vi "Circle_Setting_UI.vi"(6 "Analysis_Setting IN":T2={"PreProcess"=enum."*Algorithm*", "Parameter"=""}, 8 "error in (no error)":errorcluster, 9 "ProjectName":string, 10 "ROI List IN":refnum<vi>, 11 "Vision_Image":T11(plugin-control)) -> (0 "error out":errorcluster, 1 "Cancel?":bool, 3 "Analysis_Setting":T2={"PreProcess"=enum."*Algorithm*", "Parameter"=""})   [LabVIEW 2019]
uses:
  <vilib>/userdefined/High Color/IMAQdx.ctl
  <vilib>/vision/NI_Vision_Development_Module.lvlib
  Controls/Analysis_Type.ctl
  Controls/Analysis_Setting.ctl
  Controls/_UI Command Cluster/Circle_UI Command Cluster.ctl
  <vilib>/vision/Measure.llb/Edge Polarity.ctl
  <vilib>/vision/Measure.llb/Edge Options.ctl
  Controls/Circle/Analysis_Circle_Parameter.ctl
  Controls/V_Analysis_Type.ctl
  Ctrl/VisionProcessName.ctl
panel:
  in  "Snap?":bool
  in  "ROI Descriptor":T1
  out "Numeric":i32
  in  "Done":bool
  in  "Clamp_UI Command":T4(ring)
  in  "Cancel":bool
  in  "ClampTab":T5(tab)
  in  "Options":T8={"Search  Direction"=0, "Edge Options"={"Edge Polarity"=0, "Kernel Size"=3, "Width"=3, "Minimum Edge Strength"=10.0, "Interpolation Type"=enum."Bilinear Fixed", "Data Processing Method"=enum."Average"}, "Show Search Area"=FALSE, "Show Search Lines"=FALSE, "Show Edges Found"=FALSE, "Show Result"=TRUE, "Search Area Color"=65280, "Search Lines Color"=255, "Edge Locations Color"=16776960, "Result Color"=16711680, "Overlay Group Name"=""} {"Search  Direction" items=["Outside to Inside", "Inside to Outside"]; "Edge Options"."Edge Polarity" items=["All Edges", "Rising Edges", "Falling Edges"]; "Edge Options"."Minimum Edge Strength" format="%.2f"; "Edge Options"."Width" step=2; "Edge Options"."Kernel Size" step=2}
  in  "Circle Fit Options":T9={"Process"=enum."Get First Edge", "Step Size"=3.0, "Max Pixel Radius"=3}
  out "Fitted Circle":T10 {"Average SNR (dB)" format="%.2f"; "Average Strength" format="%.2f"; "Roundness (Real-World)" format="%.2f"; "Radius (Real-World)" format="%.2f"; "Center (Real-World)"."Y" format="%.2f"; "Center (Real-World)"."X" format="%.2f"; "Radius (Pixels)" format="%.2f"; "Center (Pixels)"."Y" format="%.2f"; "Center (Pixels)"."X" format="%.2f"}
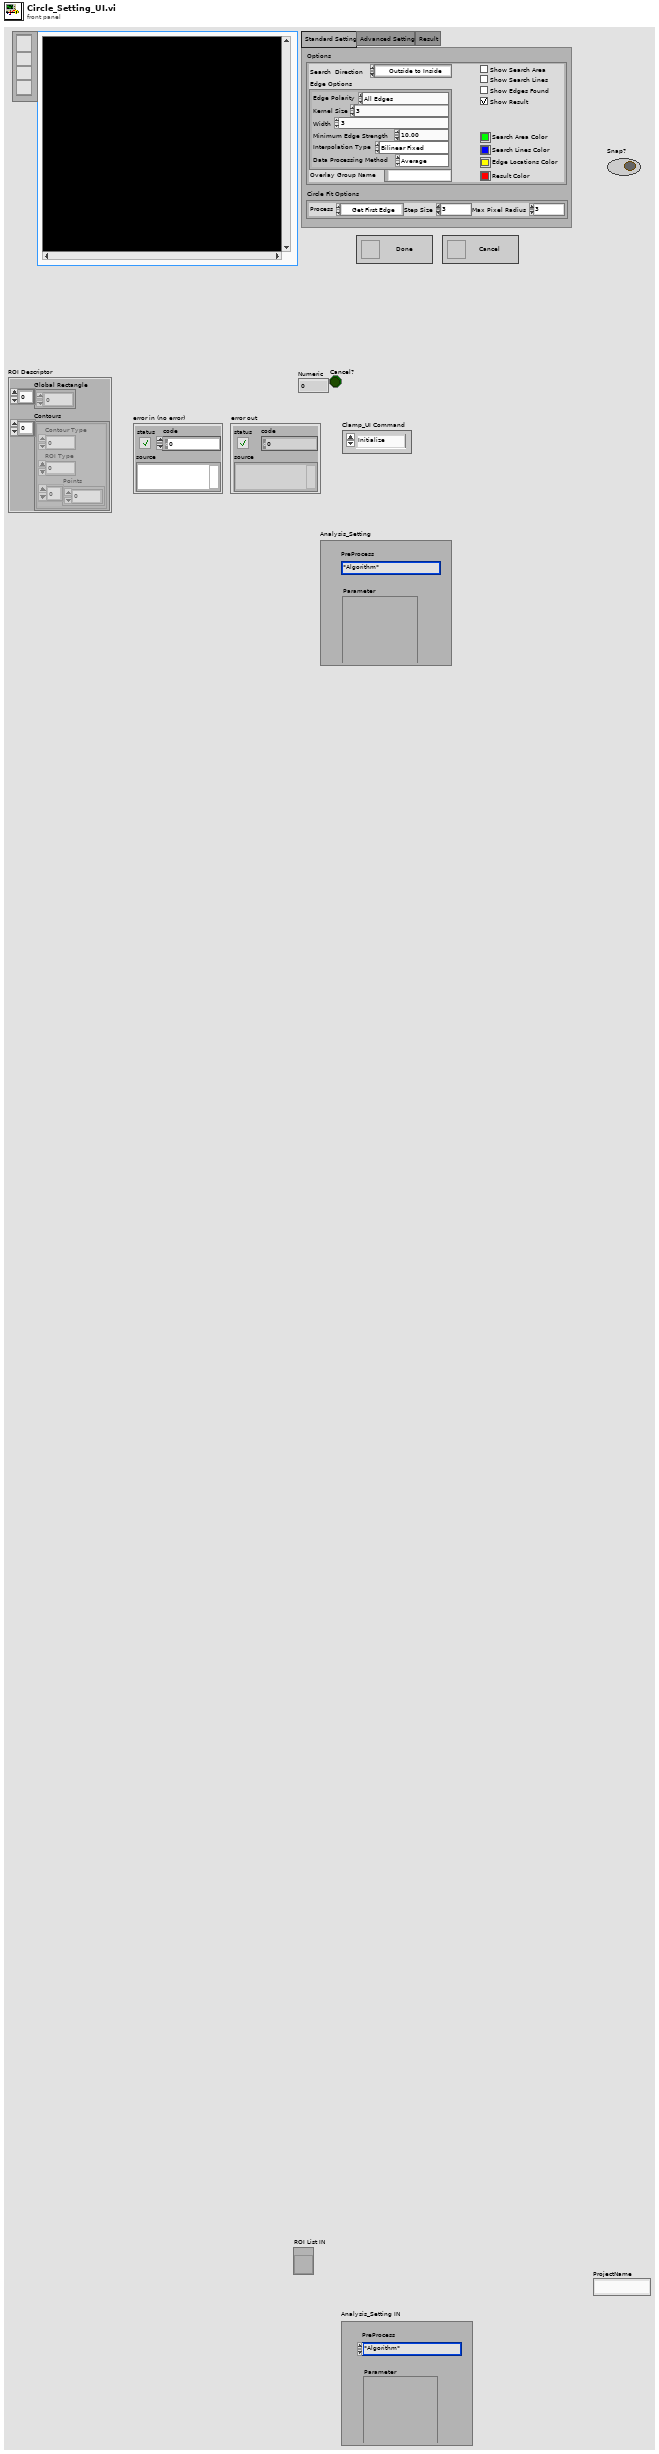
[diagram p1: front panel]
types:
  T1 = cluster{"Global Rectangle":i32[], "Contours":cluster{"Contour Type":u32, "ROI Type":u32, "Points":i32[]}[]}
  T2 = typedef "Analysis_Setting.ctl" = cluster{"PreProcess":T3, "Parameter":string}
  T3 = typedef "VisionProcessName.ctl" = enum16{"*CamParameter*", "CamAttributes", "*Preprocess*", "CG_Brightness", "C_Plane Extraction", "C_Threshold", "G_Lookup Table", "G_Threshold", "B_Image Inversion", "*Algorithm*", "CG_Histogram", "C_Color Matching", "C_Color Pattern Matching", "G_PatternMatch", "CG_Find Straight Edge", "CG_Adv. Find Straight Edge", "CG_Find Circular Edge", "G_Max Clamp", "G_Clamp (Rake)", "G_Pattern Matching"}
  T4 = enum16{"Initialize", "Done", "Run Algorithm", "Cancel"}
  T5 = enum32{"Standard Setting", "Advanced Setting", "Result"}
  T6 = typedef "Edge Options.ctl" = cluster{"Edge Polarity":T7, "Kernel Size":u32, "Width":u32, "Minimum Edge Strength":sgl, "Interpolation Type":enum32{"Zero Order", "Bilinear", "Quadratic", "Cubic", "Bilinear Fixed"}, "Data Processing Method":enum32{"Average", "Median"}}
  T7 = typedef "Edge Polarity.ctl" = u32
  T8 = cluster{"Search  Direction":u32, "Edge Options":T6, "Show Search Area":bool, "Show Search Lines":bool, "Show Edges Found":bool, "Show Result":bool, "Search Area Color":u32, "Search Lines Color":u32, "Edge Locations Color":u32, "Result Color":u32, "Overlay Group Name":string}
  T9 = cluster{"Process":enum16{"Get First Edge", "Get First + Last Edge", "Get All Edges", "Get Best Edge"}, "Step Size":dbl, "Max Pixel Radius":i32}
  T10 = cluster{"Center (Pixels)":cluster{"X":sgl, "Y":sgl}, "Radius (Pixels)":dbl, "Center (Real-World)":cluster{"X":sgl, "Y":sgl}, "Radius (Real-World)":dbl, "Roundness (Real-World)":dbl, "Average Strength":dbl, "Average SNR (dB)":dbl}
  T11 = typedef "IMAQ Image.ctl" = refnum<image>
  T12 = typedef "Circle_UI Command Cluster.ctl" = cluster{"Circle_UI Command":enum16{"Initialize", "Done", "Run Algorithm", "Cancel"}, "Snap Simulation Mouse Down":bool, "ROI Descriptor":cluster{"Global Rectangle":i32[], "Contours":cluster{"Contour Type":u32, "ROI Type":u32, "Points":i32[]}[]}, "Options":cluster{"Search  Direction":u32, "Edge Options":T6, "Show Search Area":bool, "Show Search Lines":bool, "Show Edges Found":bool, "Show Result":bool, "Search Area Color":u32, "Search Lines Color":u32, "Edge Locations Color":u32, "Result Color":u32, "Overlay Group Name":string}, "Circle Fit Options":cluster{"Process":enum16{"Get First Edge", "Get First + Last Edge", "Get All Edges", "Get Best Edge"}, "Step Size":dbl, "Max Pixel Radius":i32}}
  T13 = typedef "IMAQ Line" = cluster{"Start X":i32, "Start Y":i32, "End X":i32, "End Y":i32}
  T14 = typedef "IMAQdx.ctl" = refnum<k21>
  T15 = cluster{"Contour Type":u32, "ROI Type":u32, "Points":i32[]}
  T16 = typedef "Image Type" = u32
  T17 = typedef "Analysis_Type.ctl" = u16
  T18 = typedef "Analysis_Circle_Parameter.ctl" = cluster{"ROI Descriptor":cluster{"Global Rectangle":i32[], "Contours":cluster{"Contour Type":u32, "ROI Type":u32, "Points":i32[]}[]}, "Options":cluster{"Search  Direction":u32, "Edge Options":T6, "Show Search Area":bool, "Show Search Lines":bool, "Show Edges Found":bool, "Show Result":bool, "Search Area Color":u32, "Search Lines Color":u32, "Edge Locations Color":u32, "Result Color":u32, "Overlay Group Name":string}, "Circle Fit Options":cluster{"Process":enum16{"Get First Edge", "Get First + Last Edge", "Get All Edges", "Get Best Edge"}, "Step Size":dbl, "Max Pixel Radius":i32}}
  T19 = typedef "ROI Descriptor" = cluster{"Global Rectangle":i32[], "Contours":cluster{"ID":enum32{"External", "Internal"}, "Type":u32, "Coordinates":i32[]}[]}
  T20 = typedef "Analysis_Setting.ctl" = cluster{"PreProcess":T21, "Parameter":string}
  T21 = typedef "V_Analysis_Type.ctl" = enum16{"None", "C_Color Pattern Matching", "G_PatternMatching", "G_ShapeDectect", "G_GeometricMatch", "B_Area Check"}
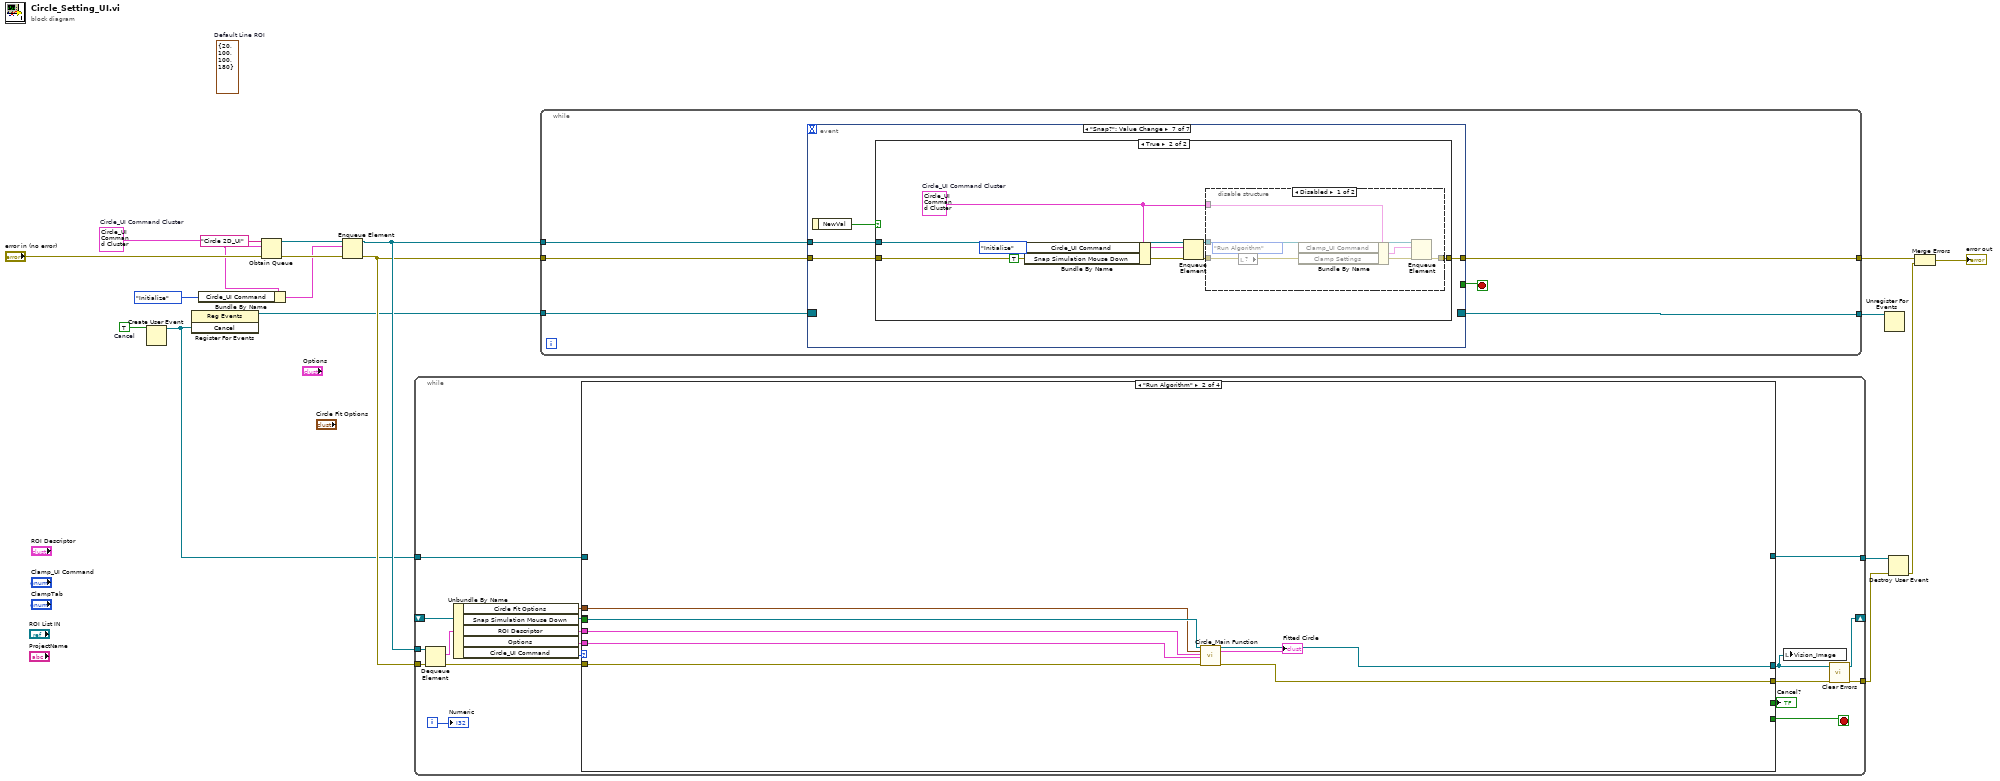
[diagram p0: block diagram]
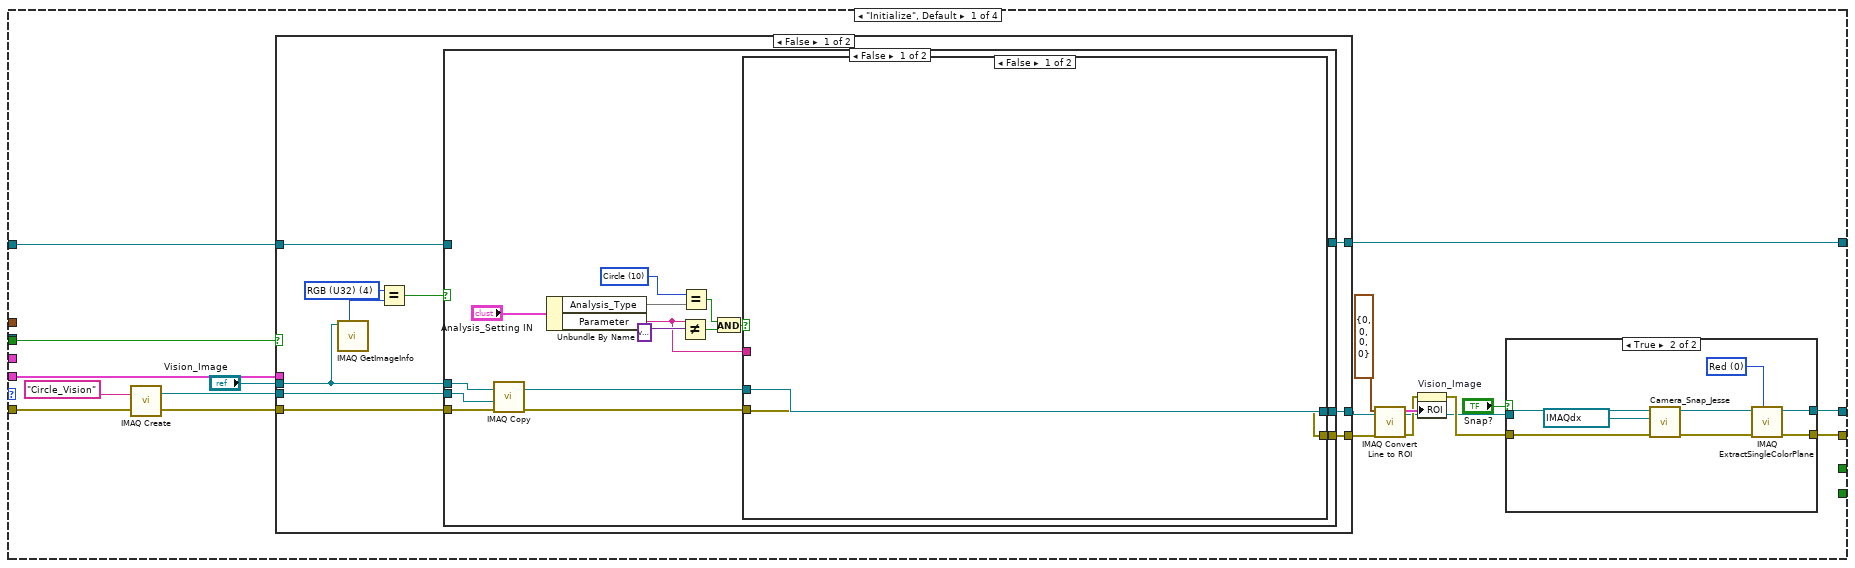
[diagram p2: hidden frame]
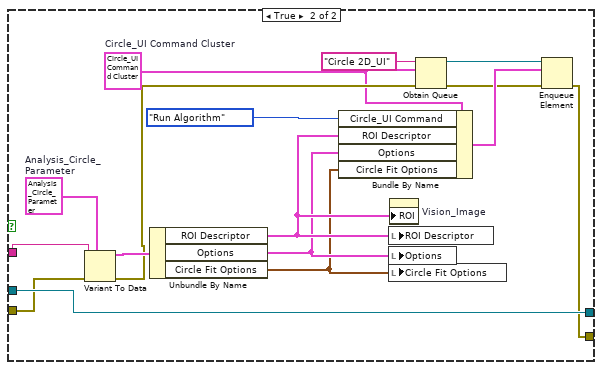
[diagram p4: hidden frame]
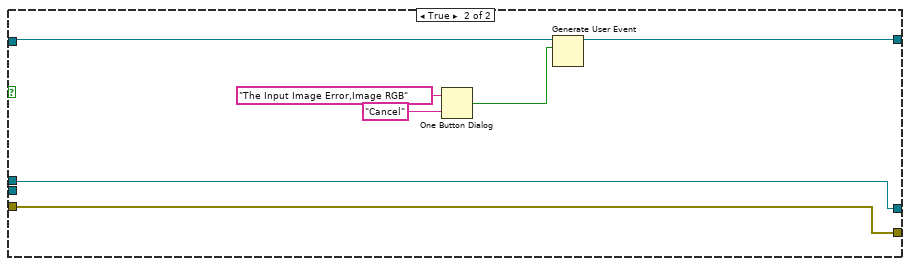
[diagram p5: hidden frame]
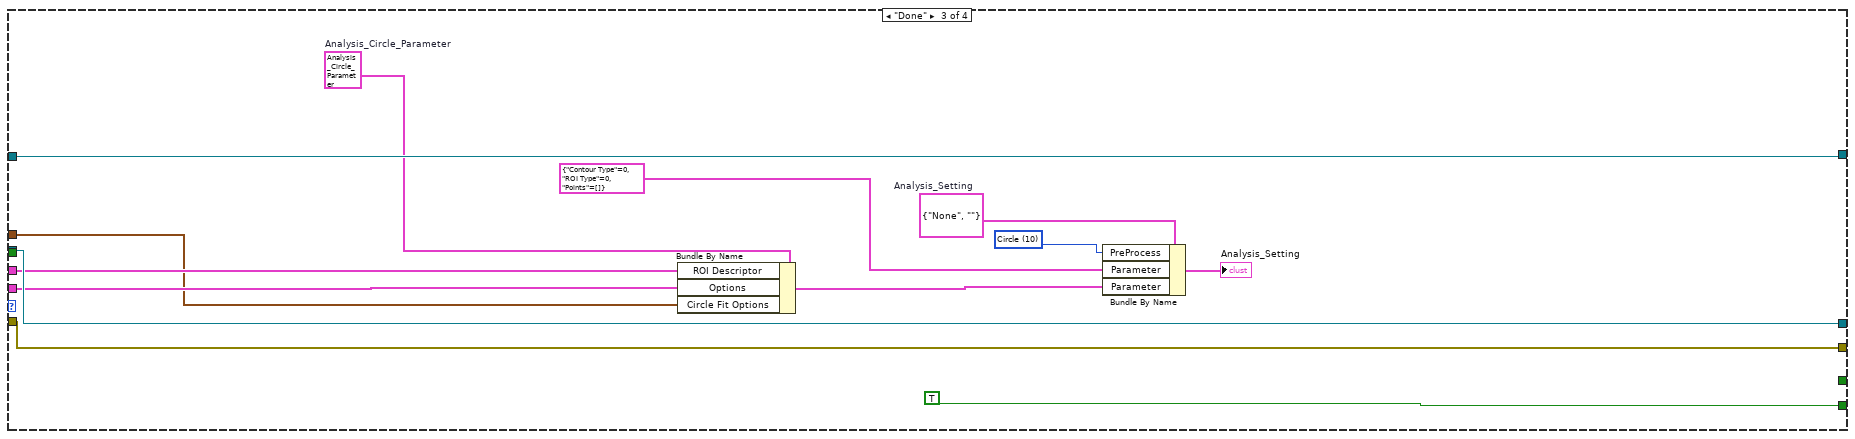
[diagram p7: hidden frame]
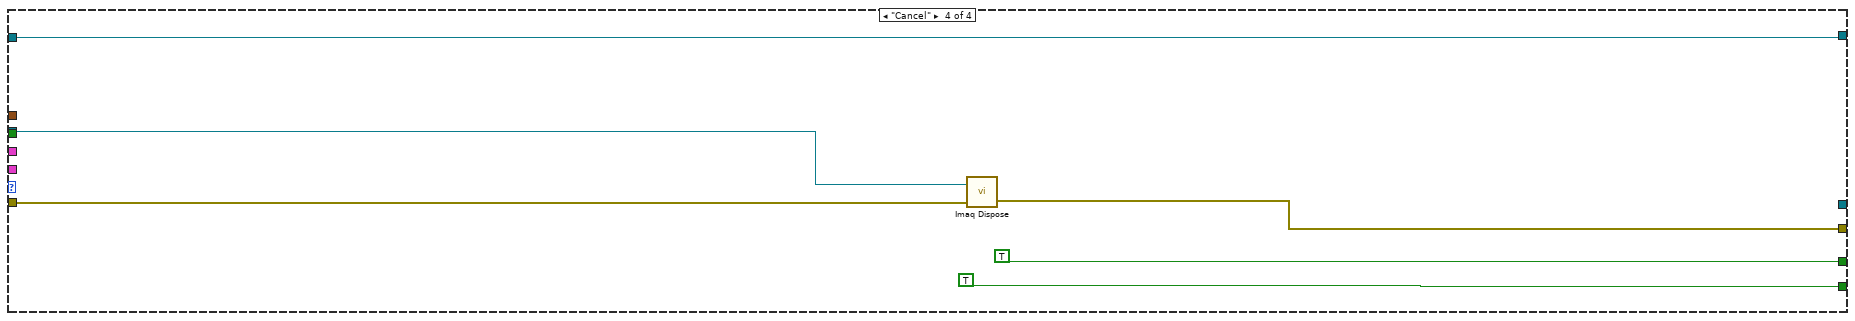
[diagram p8: hidden frame]
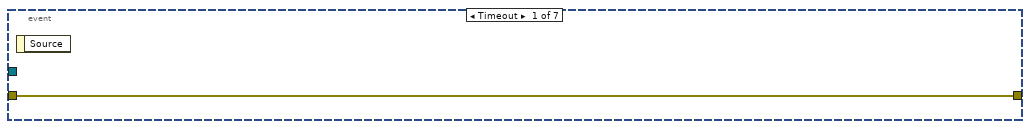
[diagram p9: hidden frame]
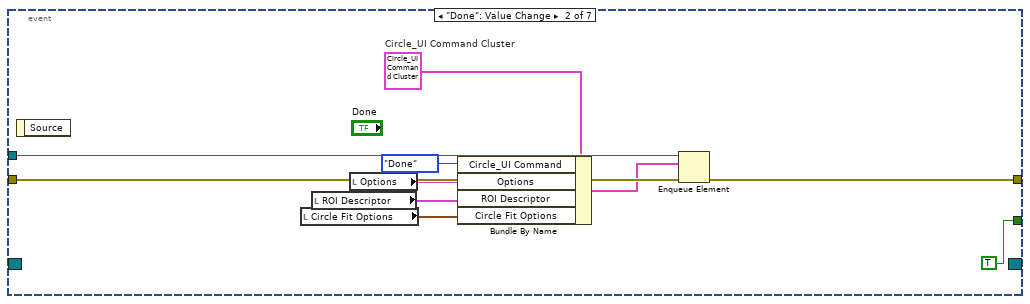
[diagram p10: hidden frame]
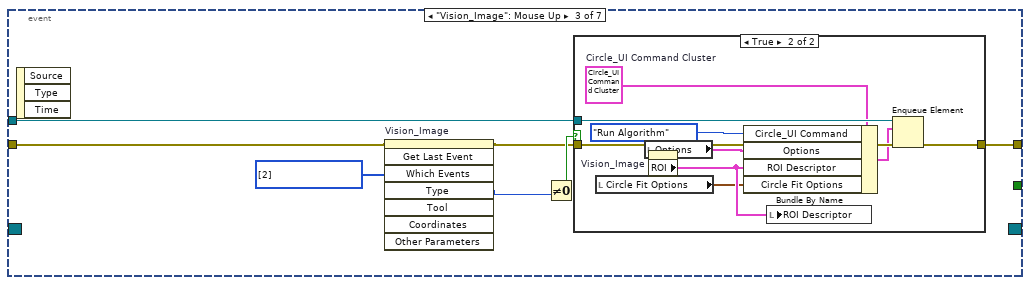
[diagram p11: hidden frame]
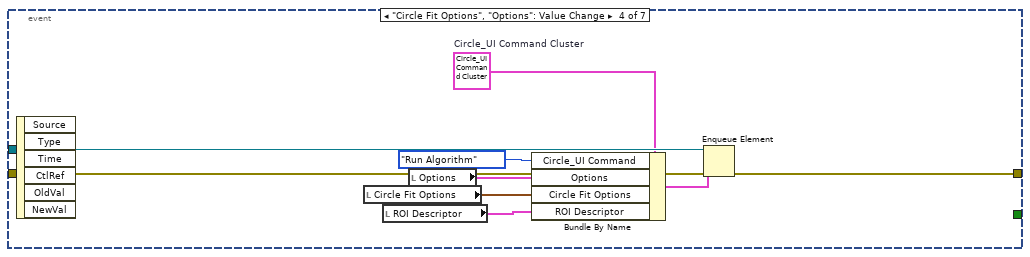
[diagram p13: hidden frame]
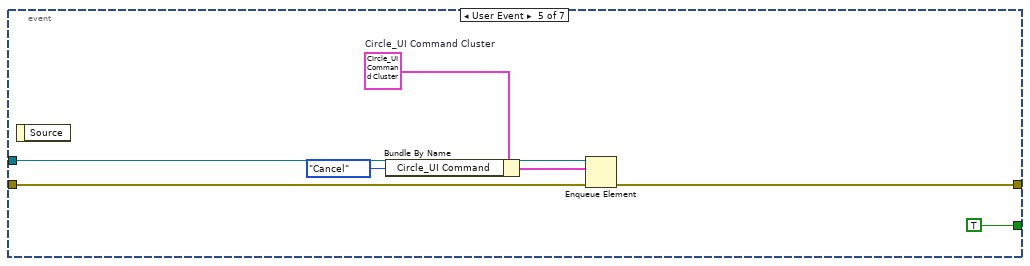
[diagram p14: hidden frame]
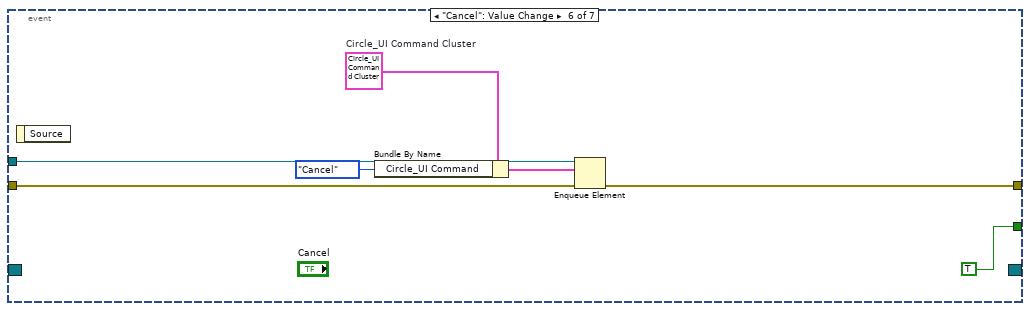
[diagram p15: hidden frame]
diagram:
  w1 = T12 {"Circle_UI Command"=enum."Initialize", "Snap Simulation Mouse Down"=FALSE, "ROI Descriptor"={"Global Rectangle"=[], "Contours"=[]}, "Options"={"Search  Direction"=40, "Edge Options"={"Edge Polarity"=0, "Kernel Size"=3, "Width"=3, "Minimum Edge Strength"=10.0, "Interpolation Type"=enum."Bilinear Fixed", "Data Processing Method"=enum."Average"}, "Show Search Area"=TRUE, "Show Search Lines"=TRUE, "Show Edges Found"=TRUE, "Show Result"=TRUE, "Search Area Color"=2, "Search Lines Color"=5, "Edge Locations Color"=4, "Result Color"=16711680, "Overlay Group Name"=""}, "Circle Fit Options"={"Process"=enum."Get First Edge", "Step Size"=3.0, "Max Pixel Radius"=3}}  # Circle_UI Command Cluster
  w8 = TRUE  # Cancel
  (unwired) T13 {"Start X"=20, "Start Y"=100, "End X"=100, "End Y"=180}  # Default Line ROI
  n1 = Create User Event(user event datatype=w8) -> (user event=w6:refnum<user-event>)  [unwired: 1 in, 1 out]
  n2 = register-events(w6) -> (reference out=w7:refnum<event-registration>)  [unwired: 2 in, 1 out]
  n3 = Bundle By Name(cluster=w1, "Circle_UI Command"=T4."Initialize" ("Barcode 2D_UI Command")) -> (w13:T12)
  n4 = Obtain Queue(name (unnamed)="Circle 2D_UI", element data type=w1, error in (no error)="error in (no error)") -> (queue out=w18:refnum<queue>, error out=w17:errorcluster)  [unwired: 2 in, 1 out]
  n5 = Enqueue Element(queue=w18, element=w13, error in (no error)=w17) -> (queue out=w12:refnum<queue>, error out=w11:errorcluster)  [unwired: 1 in, 1 out]
  n6 = while {
    tunnel: w12 -> [w36]
    tunnel: w11 -> [w35]
    shift-right: [w29] -> _
    shift-left: _ -> [w31]
    tunnel: [w20] -> w2
    tunnel: w6 -> [w23]
    tunnel: [w22] -> w4
    i -> [w30]
    stop <- w32 stop-if-true
    n7 = Dequeue Element(queue=w36, error in (no error)=w35) -> (element=w33:T12, error out=w34:errorcluster)  [unwired: 1 in, 2 out]
    n8 = Unbundle By Name(w33) -> ("Circle Fit Options"=w24:T9, "Snap Simulation Mouse Down"=w25:bool, "ROI Descriptor"=w21:T1, "Options"=w28:T8, "Circle_UI Command"=w27:T4)
    n9 = case shown="\"Run Algorithm\"" w27 {
      tunnel: w34 -> [w54 w124 w135 w141]
      tunnel: [w39 w123 w135 w140] -> w19
      tunnel: [_ _ TRUE TRUE] -> w32
      tunnel: [w40 w122 w136 _] -> w29
      tunnel: w31 -> [_ w121 w136 w142]
      tunnel: w28 -> [w51 w118 w127 _]
      tunnel: [_ _ _ TRUE] -> w26
      tunnel: w25 -> [w52 _ _ _]
      tunnel: w24 -> [_ w120 w125 _]
      tunnel: w23 -> [w38 _ w129 w138]
      tunnel: [w37 _ w129 w138] -> w22
      tunnel: w21 -> [_ w119 w126 _]
      frame "Initialize", Default {
        n10 = call "IMAQ Create"("Image Name"="Circle_Vision", "error in (no error)"=w54) -> ("New Image"=w49:T11, "error out"=w50:errorcluster)  [unwired: 3 in]
        n11 = case shown="False" w52 {
          tunnel: [w74 w116] -> w41
          tunnel: [w73 w115] -> w42
          tunnel: w51 -> [_ _]
          tunnel: w50 -> [w72 w116]
          tunnel: w49 -> [w71 w115]
          tunnel: "Vision_Image" -> [w70 _]
          tunnel: w38 -> [w66 _]
          tunnel: [w65 _] -> w37
          frame False {
            w68 = T16 4 items=["Grayscale (U8)", "Grayscale (I16)", "Grayscale (SGL)", "Complex (CSG)", "RGB (U32)", "HSL (U32)", "RGB (U64)", "Grayscale (U16)"] ("x")
            n12 = call "IMAQ GetImageInfo"("Image"=w70) -> ("Image Type"=w69:T16)  [unwired: 3 in, 7 out]
            n13 = Equal?(x=w68, y=w69) -> (x = y?=w67:bool)
            n14 = case shown="False" w67 {
              tunnel: [w89 w108] -> w74
              tunnel: [w88 w109] -> w73
              tunnel: w72 -> [w79 w108]
              tunnel: w71 -> [w78 _]
              tunnel: w70 -> [w75 w109]
              tunnel: w66 -> [_ w111]
              tunnel: [_ w110] -> w65
              frame False {
                w85 = T17 10 items=["None", "PatternMatch", "Edge Detection", "Barcode 1D", "Barcode 2D", "Clamp", "Clamp MAX", "Particle", "Histogram", "Straight Edge", "Circle", "Shape Detect", "OCR", "Contour", "ColorMatch"] ("x")
                n15 = call "IMAQ Copy"("error in (no error)"=w79, "Image Dst"=w78, "Image Src"=w75) -> ("error out"=w77:errorcluster, "Image Dst Out"=w76:T11)  [unwired: 3 in]
                n16 = Unbundle By Name("Analysis_Setting IN") -> ("Analysis_Type"=w84, "Parameter"=w80:string)
                n17 = Not Equal?(x=w80, y=variant) -> (x != y?=w86:bool)
                n18 = Equal?(x=w85, y=w84) -> (x = y?=w87:bool)
                n19 = And(x=w87, y=w86) -> (x .and. y?=w81:bool)
                n20 = case shown="False" w81 {
                  tunnel: w77 -> [w90 w98]
                  tunnel: [w90 w96] -> w89
                  tunnel: [w91 w107] -> w88
                  tunnel: w76 -> [w91 w107]
                  tunnel: w80 -> [_ w106]
                  frame False {
                  }
                  frame True {
                    w95 = T12 {"Circle_UI Command"=enum."Initialize", "Snap Simulation Mouse Down"=FALSE, "ROI Descriptor"={"Global Rectangle"=[], "Contours"=[]}, "Options"={"Search  Direction"=40, "Edge Options"={"Edge Polarity"=0, "Kernel Size"=3, "Width"=3, "Minimum Edge Strength"=10.0, "Interpolation Type"=enum."Bilinear Fixed", "Data Processing Method"=enum."Average"}, "Show Search Area"=TRUE, "Show Search Lines"=TRUE, "Show Edges Found"=TRUE, "Show Result"=TRUE, "Search Area Color"=2, "Search Lines Color"=5, "Edge Locations Color"=4, "Result Color"=16711680, "Overlay Group Name"=""}, "Circle Fit Options"={"Process"=enum."Get First Edge", "Step Size"=3.0, "Max Pixel Radius"=3}}  # Circle_UI Command Cluster
                    w105 = T18 {"ROI Descriptor"={"Global Rectangle"=[], "Contours"=[]}, "Options"={"Search  Direction"=0, "Edge Options"={"Edge Polarity"=0, "Kernel Size"=3, "Width"=3, "Minimum Edge Strength"=10.0, "Interpolation Type"=enum."Bilinear Fixed", "Data Processing Method"=enum."Average"}, "Show Search Area"=FALSE, "Show Search Lines"=FALSE, "Show Edges Found"=FALSE, "Show Result"=TRUE, "Search Area Color"=65280, "Search Lines Color"=255, "Edge Locations Color"=16776960, "Result Color"=16711680, "Overlay Group Name"=""}, "Circle Fit Options"={"Process"=enum."Get First Edge", "Step Size"=3.0, "Max Pixel Radius"=3}}  # Analysis_Circle_Parameter
                    n21 = Variant To Data(error in=w98, type=w105, Variant=w106) -> (data=w104:T18, error out=w97:errorcluster)
                    n22 = Unbundle By Name(w104) -> ("ROI Descriptor"=w94:T1, "Options"=w93:T8, "Circle Fit Options"=w92:T9)
                    n23 = Bundle By Name(cluster=w95, "Circle_UI Command"=T4."Run Algorithm" ("Barcode 2D_UI Command"), "ROI Descriptor"=w94, "Options"=w93, "Circle Fit Options"=w92) -> (w103:T12)
                    n24 = local write "ROI Descriptor"(w94) -> ()
                    n25 = local write "Options"(w93) -> ()
                    n26 = local write "Circle Fit Options"(w92) -> ()
                    n27 = property on="Vision_Image" class="ImageControl"("ROI"=w94) -> ()  [unwired: 2 in, 2 out]
                    n28 = Obtain Queue(name (unnamed)="Circle 2D_UI", element data type=w95, error in (no error)=w97) -> (queue out=w99:refnum<queue>, error out=w100:errorcluster)  [unwired: 2 in, 1 out]
                    n29 = Enqueue Element(queue=w99, element=w103, error in (no error)=w100) -> (error out=w96:errorcluster)  [unwired: 1 in, 2 out]
                  }
                }
              }
              frame True {
                n30 = One Button Dialog(message="The Input Image Error,Image RGB", button name ("OK")="Cancel") -> (true=w112:bool)
                n31 = Generate User Event(user event=w111, event data cluster=w112) -> (user event out=w110:refnum<user-event>)  [unwired: 2 in, 1 out]
              }
            }
          }
          frame True {
          }
        }
        n32 = call "IMAQ Convert Line to ROI"("error in (no error)"=w41, "Line"=T13 {"Start X"=0, "Start Y"=0, "End X"=0, "End Y"=0}) -> ("error out"=w44:errorcluster, "ROI Descriptor"=w45:T19)  [unwired: 7 in]
        n33 = property on="Vision_Image" class="ImageControl"(error in=w44, "ROI"=w45) -> (error out=w43:errorcluster)  [unwired: 1 in, 1 out]
        n34 = case shown="True" "Snap?" {
          tunnel: [w56 w60] -> w39
          tunnel: [w55 w59] -> w40
          tunnel: w43 -> [w56 w57]
          tunnel: w42 -> [w55 w58]
          frame False {
          }
          frame True {
            w62 = 0 items=["Red", "Green", "Blue", "Hue", "Saturation", "Luminance", "Value", "Intensity"] ("Color Plane")
            n35 = call "Camera_Snap_Jesse.vi"("error in (no error)"=w57, "Camera Session In"=T14 "cam01", "Image In"=w58) -> ("error out"=w61:errorcluster, "New Image"=w63:T11)  [unwired: 7 in]
            n36 = call "IMAQ ExtractSingleColorPlane"("Color Plane"=w62, "error in (no error)"=w61, "Image Src"=w63) -> ("error out"=w60:errorcluster, "Image Dst Out"=w59:T11)  [unwired: 1 in, 6 out]
          }
        }
      }
      frame "Run Algorithm" {
        n37 = call "Circle_Main Function.vi"("Refnum in"=w121, "Circle Fit Options"=w120, "ROI"=w119, "Options"=w118, "error in (no error)"=w124) -> ("Refnum out"=w122:T11, "Fitted Circle"=→"Fitted Circle":T10, "error out"=w123:errorcluster)  [unwired: 12 in]
      }
      frame "Done" {
        w128 = T18 {"ROI Descriptor"={"Global Rectangle"=[], "Contours"=[]}, "Options"={"Search  Direction"=0, "Edge Options"={"Edge Polarity"=0, "Kernel Size"=3, "Width"=3, "Minimum Edge Strength"=10.0, "Interpolation Type"=enum."Bilinear Fixed", "Data Processing Method"=enum."Average"}, "Show Search Area"=FALSE, "Show Search Lines"=FALSE, "Show Edges Found"=FALSE, "Show Result"=TRUE, "Search Area Color"=65280, "Search Lines Color"=255, "Edge Locations Color"=16776960, "Result Color"=16711680, "Overlay Group Name"=""}, "Circle Fit Options"={"Process"=enum."Get First Edge", "Step Size"=3.0, "Max Pixel Radius"=3}}  # Analysis_Circle_Parameter
        w133 = T17 10 items=["None", "PatternMatch", "Edge Detection", "Barcode 1D", "Barcode 2D", "Clamp", "Clamp MAX", "Particle", "Histogram", "Straight Edge", "Circle", "Shape Detect", "OCR", "Contour", "ColorMatch"] ("Analysis_Type")
        w134 = T20 {"PreProcess"=enum."None", "Parameter"=""}  # Analysis_Setting
        n38 = Bundle By Name(cluster=w128, "ROI Descriptor"=w126, "Options"=w127, "Circle Fit Options"=w125) -> (w131:T18)
        n39 = Bundle By Name(cluster=w134, "PreProcess"=w133, "Parameter"=T15 {"Contour Type"=0, "ROI Type"=0, "Points"=[]} ("RegionContour"), "Parameter"=w131) -> (→"Analysis_Setting":T20)
      }
      frame "Cancel" {
        n40 = call "Imaq Dispose"("Image"=w142, "error in (no error)"=w141) -> ("error out"=w140:errorcluster)  [unwired: 4 in]
      }
    }
    "Cancel?" <- w26
    n41 = local write "Vision_Image"(w29) -> ()
    n42 = call <vilib>:"Clear Errors.vi"("error in (no error)"=w19) -> ("error out"=w20:errorcluster)  [unwired: 5 in, 1 out]
    "Numeric" <- w30
  }
  n43 = while {
    tunnel: w12 -> [w149]
    tunnel: w11 -> [w148]
    tunnel: [w146] -> w15
    tunnel: w7 -> [w145]
    tunnel: [w144] -> w5
    stop <- w147 stop-if-true
    n44 = event shown="[6] \"Snap?\": Value Change" {
      selector: w145 -> [_ _ _ _ _ _ _]
      dyn-events: [_ _ _ _ _ _ _] -> w144
      timeout: _ -> [_ _ _ _ _ _ _]
      tunnel: w149 -> [_ w160 w167 w186 w191 w200 w203]
      tunnel: w148 -> [w150 w159 w164 w185 w190 w199 w202]
      tunnel: [_ TRUE _ _ TRUE TRUE _] -> w147
      tunnel: [w150 w158 w161 w184 w187 w197 w201] -> w146
      event Timeout {
        n45 = event-data() -> ()  [unwired: 1 in, 1 out]
      }
      event "Done": Value Change {
        w153 = T12 {"Circle_UI Command"=enum."Initialize", "Snap Simulation Mouse Down"=FALSE, "ROI Descriptor"={"Global Rectangle"=[], "Contours"=[]}, "Options"={"Search  Direction"=40, "Edge Options"={"Edge Polarity"=0, "Kernel Size"=3, "Width"=3, "Minimum Edge Strength"=10.0, "Interpolation Type"=enum."Bilinear Fixed", "Data Processing Method"=enum."Average"}, "Show Search Area"=TRUE, "Show Search Lines"=TRUE, "Show Edges Found"=TRUE, "Show Result"=TRUE, "Search Area Color"=2, "Search Lines Color"=5, "Edge Locations Color"=4, "Result Color"=16711680, "Overlay Group Name"=""}, "Circle Fit Options"={"Process"=enum."Get First Edge", "Step Size"=3.0, "Max Pixel Radius"=3}}  # Circle_UI Command Cluster
        n46 = event-data() -> ()  [unwired: 1 in, 1 out]
        n47 = local read "Circle Fit Options"() -> (w151:T9)
        n48 = local read "ROI Descriptor"() -> (w154:T1)
        n49 = local read "Options"() -> (w152:T8)
        n50 = Bundle By Name(cluster=w153, "Circle_UI Command"=T4."Done" ("Edge Detection_UI Command"), "Options"=w152, "ROI Descriptor"=w154, "Circle Fit Options"=w151) -> (w156:T12)
        n51 = Enqueue Element(queue=w160, element=w156, error in (no error)=w159) -> (error out=w158:errorcluster)  [unwired: 1 in, 2 out]
      }
      event "Vision_Image": Mouse Up {
        w165 = i32[] [2] items=["No Event"=0, "Click Event"=1, "Draw Event"=2, "Size Event"=4, "Scroll Event"=5, "Double Click Event"=8] ("Which Events")
        n52 = event-data() -> ()  [unwired: 1 in, 3 out]
        n53 = invoke on="Vision_Image" class="ImageControl" method="Get Last Event"(error in=w164, "Which Events"=w165) -> (error out=w163:errorcluster, "Type"=w162:i32)  [unwired: 6 in, 6 out]
        n54 = Not Equal To 0?(x=w162) -> (x != 0?=w166:bool)
        n55 = case shown="True" w166 {
          tunnel: w167 -> [_ w177]
          tunnel: w163 -> [w168 w176]
          tunnel: [w168 w173] -> w161
          frame False {
          }
          frame True {
            w171 = T12 {"Circle_UI Command"=enum."Initialize", "Snap Simulation Mouse Down"=FALSE, "ROI Descriptor"={"Global Rectangle"=[], "Contours"=[]}, "Options"={"Search  Direction"=40, "Edge Options"={"Edge Polarity"=0, "Kernel Size"=3, "Width"=3, "Minimum Edge Strength"=10.0, "Interpolation Type"=enum."Bilinear Fixed", "Data Processing Method"=enum."Average"}, "Show Search Area"=TRUE, "Show Search Lines"=TRUE, "Show Edges Found"=TRUE, "Show Result"=TRUE, "Search Area Color"=2, "Search Lines Color"=5, "Edge Locations Color"=4, "Result Color"=16711680, "Overlay Group Name"=""}, "Circle Fit Options"={"Process"=enum."Get First Edge", "Step Size"=3.0, "Max Pixel Radius"=3}}  # Circle_UI Command Cluster
            n56 = local read "Circle Fit Options"() -> (w169:T9)
            n57 = local read "Options"() -> (w170:T8)
            n58 = property on="Vision_Image" class="ImageControl"() -> ("ROI"=w172:T1)  [unwired: 2 in, 2 out]
            n59 = Bundle By Name(cluster=w171, "Circle_UI Command"=T4."Run Algorithm" ("Clamp_UI Command"), "Options"=w170, "ROI Descriptor"=w172, "Circle Fit Options"=w169) -> (w174:T12)
            n60 = local write "ROI Descriptor"(w172) -> ()
            n61 = Enqueue Element(queue=w177, element=w174, error in (no error)=w176) -> (error out=w173:errorcluster)  [unwired: 1 in, 2 out]
          }
        }
      }
      event "Circle Fit Options", "Options": Value Change {
        w180 = T12 {"Circle_UI Command"=enum."Initialize", "Snap Simulation Mouse Down"=FALSE, "ROI Descriptor"={"Global Rectangle"=[], "Contours"=[]}, "Options"={"Search  Direction"=40, "Edge Options"={"Edge Polarity"=0, "Kernel Size"=3, "Width"=3, "Minimum Edge Strength"=10.0, "Interpolation Type"=enum."Bilinear Fixed", "Data Processing Method"=enum."Average"}, "Show Search Area"=TRUE, "Show Search Lines"=TRUE, "Show Edges Found"=TRUE, "Show Result"=TRUE, "Search Area Color"=2, "Search Lines Color"=5, "Edge Locations Color"=4, "Result Color"=16711680, "Overlay Group Name"=""}, "Circle Fit Options"={"Process"=enum."Get First Edge", "Step Size"=3.0, "Max Pixel Radius"=3}}  # Circle_UI Command Cluster
        n62 = event-data() -> ()  [unwired: 1 in, 6 out]
        n63 = local read "Circle Fit Options"() -> (w178:T9)
        n64 = local read "ROI Descriptor"() -> (w181:T1)
        n65 = local read "Options"() -> (w179:T8)
        n66 = Bundle By Name(cluster=w180, "Circle_UI Command"=T4."Run Algorithm" ("Barcode 2D_UI Command"), "Options"=w179, "Circle Fit Options"=w178, "ROI Descriptor"=w181) -> (w183:T12)
        n67 = Enqueue Element(queue=w186, element=w183, error in (no error)=w185) -> (error out=w184:errorcluster)  [unwired: 1 in, 2 out]
      }
      event User Event {
        w188 = T12 {"Circle_UI Command"=enum."Initialize", "Snap Simulation Mouse Down"=FALSE, "ROI Descriptor"={"Global Rectangle"=[], "Contours"=[]}, "Options"={"Search  Direction"=40, "Edge Options"={"Edge Polarity"=0, "Kernel Size"=3, "Width"=3, "Minimum Edge Strength"=10.0, "Interpolation Type"=enum."Bilinear Fixed", "Data Processing Method"=enum."Average"}, "Show Search Area"=TRUE, "Show Search Lines"=TRUE, "Show Edges Found"=TRUE, "Show Result"=TRUE, "Search Area Color"=2, "Search Lines Color"=5, "Edge Locations Color"=4, "Result Color"=16711680, "Overlay Group Name"=""}, "Circle Fit Options"={"Process"=enum."Get First Edge", "Step Size"=3.0, "Max Pixel Radius"=3}}  # Circle_UI Command Cluster
        n68 = event-data() -> ()  [unwired: 1 in, 1 out]
        n69 = Bundle By Name(cluster=w188, "Circle_UI Command"=T4."Cancel" ("Barcode 1D_UI Command")) -> (w192:T12)
        n70 = Enqueue Element(queue=w191, element=w192, error in (no error)=w190) -> (error out=w187:errorcluster)  [unwired: 1 in, 2 out]
      }
      event "Cancel": Value Change {
        w194 = T12 {"Circle_UI Command"=enum."Initialize", "Snap Simulation Mouse Down"=FALSE, "ROI Descriptor"={"Global Rectangle"=[], "Contours"=[]}, "Options"={"Search  Direction"=40, "Edge Options"={"Edge Polarity"=0, "Kernel Size"=3, "Width"=3, "Minimum Edge Strength"=10.0, "Interpolation Type"=enum."Bilinear Fixed", "Data Processing Method"=enum."Average"}, "Show Search Area"=TRUE, "Show Search Lines"=TRUE, "Show Edges Found"=TRUE, "Show Result"=TRUE, "Search Area Color"=2, "Search Lines Color"=5, "Edge Locations Color"=4, "Result Color"=16711680, "Overlay Group Name"=""}, "Circle Fit Options"={"Process"=enum."Get First Edge", "Step Size"=3.0, "Max Pixel Radius"=3}}  # Circle_UI Command Cluster
        n71 = event-data() -> ()  [unwired: 1 in, 1 out]
        n72 = Bundle By Name(cluster=w194, "Circle_UI Command"=T4."Cancel" ("Barcode 1D_UI Command")) -> (w195:T12)
        n73 = Enqueue Element(queue=w200, element=w195, error in (no error)=w199) -> (error out=w197:errorcluster)  [unwired: 1 in, 2 out]
      }
      event "Snap?": Value Change {
        n74 = event-data() -> ("NewVal"=w204:bool)  [unwired: 1 in]
        n75 = case shown="True" w204 {
          tunnel: w203 -> [_ w214]
          tunnel: w202 -> [w205 w213]
          tunnel: [w205 w209] -> w201
          frame False {
          }
          frame True {
            w206 = T12 {"Circle_UI Command"=enum."Initialize", "Snap Simulation Mouse Down"=FALSE, "ROI Descriptor"={"Global Rectangle"=[], "Contours"=[]}, "Options"={"Search  Direction"=40, "Edge Options"={"Edge Polarity"=0, "Kernel Size"=3, "Width"=3, "Minimum Edge Strength"=10.0, "Interpolation Type"=enum."Bilinear Fixed", "Data Processing Method"=enum."Average"}, "Show Search Area"=TRUE, "Show Search Lines"=TRUE, "Show Edges Found"=TRUE, "Show Result"=TRUE, "Search Area Color"=2, "Search Lines Color"=5, "Edge Locations Color"=4, "Result Color"=16711680, "Overlay Group Name"=""}, "Circle Fit Options"={"Process"=enum."Get First Edge", "Step Size"=3.0, "Max Pixel Radius"=3}}  # Circle_UI Command Cluster
            n76 = Bundle By Name(cluster=w206, "Circle_UI Command"=T4."Initialize" ("Barcode 2D_UI Command"), "Snap Simulation Mouse Down"=TRUE) -> (w208:T12)
            n77 = Enqueue Element(queue=w214, element=w208, error in (no error)=w213) -> (queue out=w211:refnum<queue>, error out=w210:errorcluster)  [unwired: 1 in, 1 out]
            n78 = disable-structure shown="Disabled" {
              disable-tunnel: w211 -> [w221 _]
              disable-tunnel: w210 -> [w220 _]
              disable-tunnel: w206 -> [w219 _]
              disable-tunnel: [w217 _] -> w209
              frame Disabled {
                n79 = local read item#-1() -> (w215)
                n80 = Bundle By Name(cluster=w219, "Clamp_UI Command"=T4."Run Algorithm" ("Barcode 2D_UI Command"), "Clamp Settings"=w215) -> (w216:T12)
                n81 = Enqueue Element(queue=w221, element=w216, error in (no error)=w220) -> (error out=w217:errorcluster)  [unwired: 1 in, 2 out]
              }
              frame Enabled {
              }
            }
          }
        }
      }
    }
  }
  n82 = Unregister For Events(event registration refnum=w5) -> ()  [unwired: 1 in, 1 out]
  n83 = Destroy User Event(user event=w4, error in=w2) -> (error out=w3:errorcluster)
  n84 = Merge Errors(w15, w3) -> (→"error out":errorcluster)
